vi "ROS_Master_getSystemStateReply.vi"(3 "ROS_Master in":T1) -> (0 "XML":string)   [LabVIEW 2014]
doc: "Returns XML for the system state reply"
uses:
  <userlib>/ROS for LabVIEW Software/ROS/Code/ROS_Master/ROS_Master.ctl
  <userlib>/ROS for LabVIEW Software/ROS/Code/ROS_Master/ROS_Topic.ctl
  <userlib>/ROS for LabVIEW Software/ROS/Code/ROS_Master/ROS_Node.ctl
  <userlib>/ROS for LabVIEW Software/ROS/Code/ROS_Master/ROS_Service.ctl
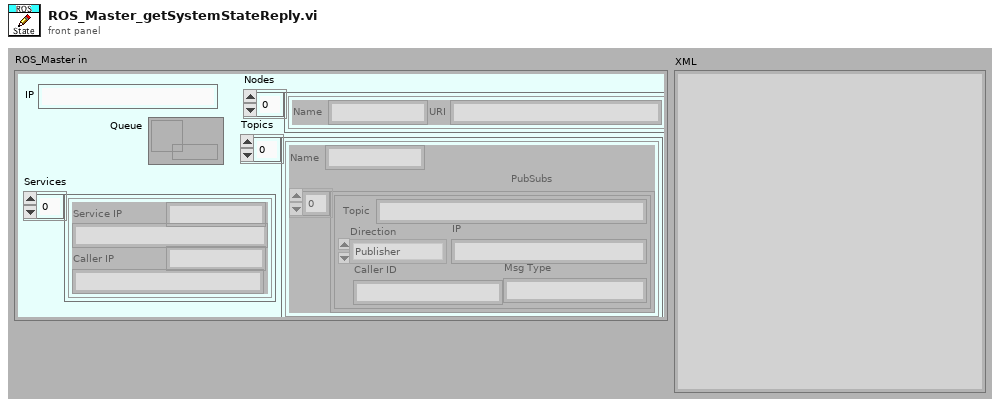
[diagram p1: front panel]
types:
  T1 = typedef "ROS_Master.ctl" = cluster{"IP":string, "Topics":cluster{"Name":string, "PubSubs":T2[]}[], "Nodes":T3[], "Services":T4[], "Queue":refnum<queue>}
  T2 = typedef "ROS_Topic.ctl" = cluster{"Caller ID":string, "IP":string, "Msg Type":string, "Direction":enum16{"Publisher", "Subscriber"}, "Topic":string}
  T3 = typedef "ROS_Node.ctl" = cluster{"Name":string, "URI":string}
  T4 = typedef "ROS_Service.ctl" = cluster{"Service":string, "Service IP":string, "Caller IP":string, "Caller ID":string}
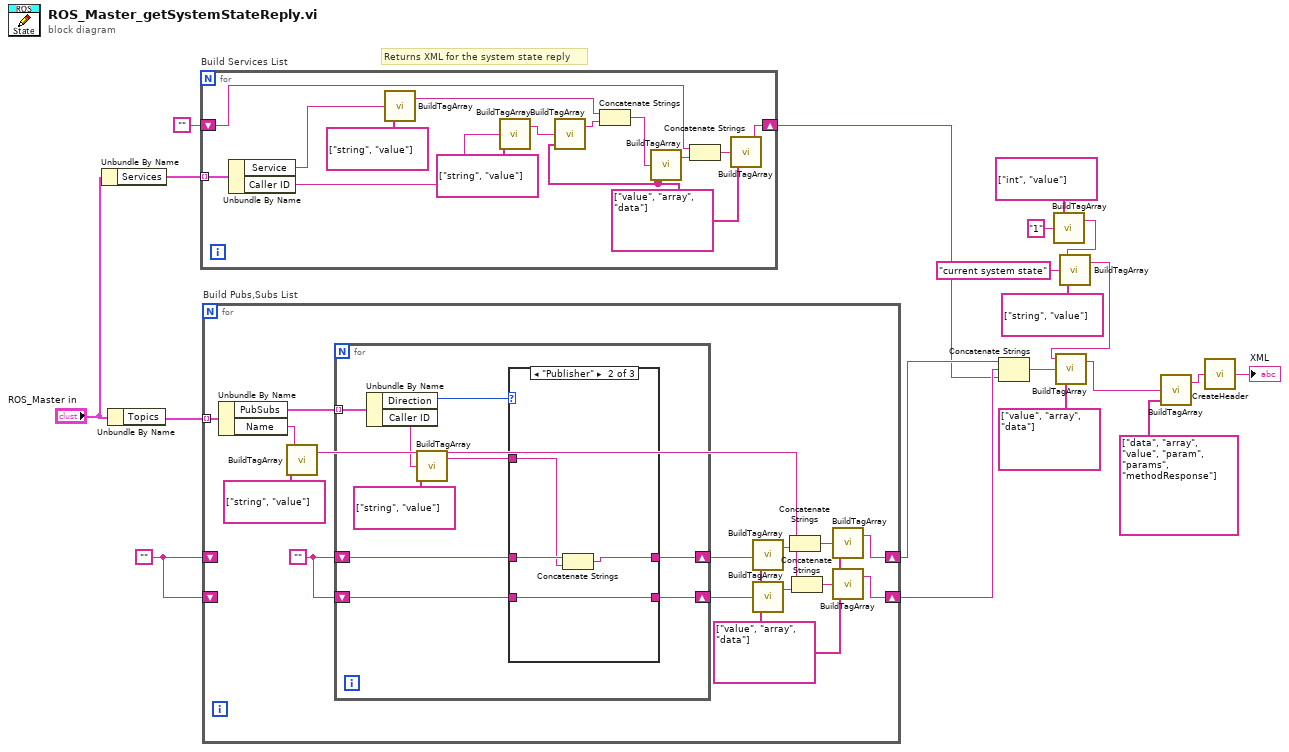
[diagram p0: block diagram]
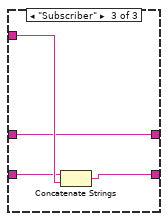
[diagram p3: hidden frame]
diagram:
  w19 = ""
  # "Returns XML for the system state reply"
  n1 = Unbundle By Name("ROS_Master in") -> ("Services"=w18:T4[])
  n2 = Unbundle By Name("ROS_Master in") -> ("Topics"=w20:cluster{"Name":string, "PubSubs":T2[]}[])
  n3 = for "Build Services List" {
    tunnel: w18 -> [w34] mode=indexing
    shift-right: [w21] -> w14
    shift-left: "" -> [w22]
    w27 = string[] ["value", "array", "data"] ("tags")
    n4 = Unbundle By Name(w34) -> ("Service"=w29:string, "Caller ID"=w28:string)
    n5 = call <userlib>:"BuildTagArray.vi"("tags"=string[] ["string", "value"], "value"=w29) -> ("string out"=w24:string)  [unwired: 2 in]
    n6 = call <userlib>:"BuildTagArray.vi"("tags"=string[] ["string", "value"], "value"=w28) -> ("string out"=w26:string)  [unwired: 2 in]
    n7 = call <userlib>:"BuildTagArray.vi"("tags"=w27, "value"=w26) -> ("string out"=w25:string)  [unwired: 2 in]
    n8 = Concatenate Strings(w24, w25) -> (w23:string)
    n9 = call <userlib>:"BuildTagArray.vi"("tags"=w27, "value"=w23) -> ("string out"=w32:string)  [unwired: 2 in]
    n10 = Concatenate Strings(w22, w32) -> (w31:string)
    n11 = call <userlib>:"BuildTagArray.vi"("tags"=w27, "value"=w31) -> ("string out"=w21:string)  [unwired: 2 in]
  }
  n12 = for "Build Pubs,Subs List" {
    tunnel: w20 -> [w49] mode=indexing
    shift-right: [w35] -> w16
    shift-left: w19 -> [_]
    shift-right: [w36] -> w15
    shift-left: w19 -> [_]
    w37 = string[] ["value", "array", "data"] ("tags")
    w45 = ""
    n13 = Unbundle By Name(w49) -> ("PubSubs"=w48:T2[], "Name"=w47:string)
    n14 = call <userlib>:"BuildTagArray.vi"("tags"=string[] ["string", "value"], "value"=w47) -> ("string out"=w39:string)  [unwired: 2 in]
    n15 = for {
      tunnel: w48 -> [w58] mode=indexing
      shift-right: [w51] -> w44
      shift-left: w45 -> [w53]
      shift-right: [w50] -> w43
      shift-left: w45 -> [w52]
      n16 = Unbundle By Name(w58) -> ("Direction"=w57:enum16{"Publisher", "Subscriber"}, "Caller ID"=w55:string)
      n17 = call <userlib>:"BuildTagArray.vi"("tags"=string[] ["string", "value"], "value"=w55) -> ("string out"=w54:string)  [unwired: 2 in]
      n18 = case shown="\"Publisher\"" w57 {
        tunnel: w54 -> [_ w63 w68]
        tunnel: w53 -> [w60 w64 w65]
        tunnel: w52 -> [w59 w61 w67]
        tunnel: [w60 w62 w65] -> w51
        tunnel: [w59 w61 w66] -> w50
        frame Default {
        }
        frame "Publisher" {
          n19 = Concatenate Strings(w64, w63) -> (w62:string)
        }
        frame "Subscriber" {
          n20 = Concatenate Strings(w67, w68) -> (w66:string)
        }
      }
    }
    n21 = call <userlib>:"BuildTagArray.vi"("tags"=w37, "value"=w44) -> ("string out"=w42:string)  [unwired: 2 in]
    n22 = call <userlib>:"BuildTagArray.vi"("tags"=w37, "value"=w43) -> ("string out"=w40:string)  [unwired: 2 in]
    n23 = Concatenate Strings(w39, w42) -> (w41:string)
    n24 = Concatenate Strings(w39, w40) -> (w38:string)
    n25 = call <userlib>:"BuildTagArray.vi"("tags"=w37, "value"=w41) -> ("string out"=w35:string)  [unwired: 2 in]
    n26 = call <userlib>:"BuildTagArray.vi"("tags"=w37, "value"=w38) -> ("string out"=w36:string)  [unwired: 2 in]
  }
  n27 = Concatenate Strings(w16, w15, w14) -> (w13:string)
  n28 = call <userlib>:"BuildTagArray.vi"("tags"=string[] ["int", "value"], "value"="1") -> ("string out"=w11:string)  [unwired: 2 in]
  n29 = call <userlib>:"BuildTagArray.vi"("tags"=string[] ["string", "value"], "value"="current system state", "string in"=w11) -> ("string out"=w7:string)  [unwired: 1 in]
  n30 = call <userlib>:"BuildTagArray.vi"("tags"=string[] ["value", "array", "data"], "value"=w13, "string in"=w7) -> ("string out"=w3:string)  [unwired: 1 in]
  n31 = call <userlib>:"BuildTagArray.vi"("tags"=string[] ["data", "array", "value", "param", "params", "methodResponse"], "value"=w3) -> ("string out"=w5:string)  [unwired: 2 in]
  n32 = call <userlib>:"CreateHeader.vi"("Content"=w5) -> ("XML"=→"XML":string)
